vi "testpy.vi"() -> ()   [LabVIEW 2018]
uses:
  <vilib>/Enthought/Python Integration Toolkit/api/Unpack Double.vi
  <vilib>/Enthought/Python Integration Toolkit/Python Integration Toolkit.lvlib
panel:
  out "Value":dbl
  in  "Numeric":dbl format="%#_13g"
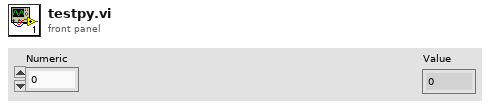
[diagram p1: front panel]
types:
  T1 = typedef "Python Integration Toolkit.lvlib/Session ID.ctl" = u64
  T2 = typedef "Python Integration Toolkit.lvlib/Python Objects.ctl" = variant
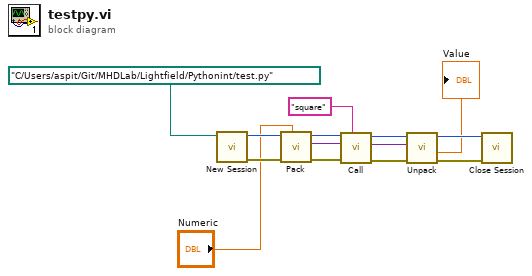
[diagram p0: block diagram]
diagram:
  n1 = call <vilib>:"New Session.vi"("Path to Python Module (.py File)"=path "C:/Users/aspit/Git/MHDLab/Lightfield/Pythonint/test.py") -> ("error out"=w10:errorcluster, "Session ID out"=w14:T1)  [unwired: 9 in]
  n2 = call <vilib>:"Pack.vi"("Argument"="Numeric", "error in (no error)"=w10, "Session ID"=w14) -> ("error out"=w9:errorcluster, "Python Object References Out"=w3:T2, "Session ID out"=w13:T1)  [unwired: 6 in]
  n3 = call <vilib>:"Call.vi"("Function or Method Name"="square", "error in (no error)"=w9, "Python Object References In"=w3, "Session ID"=w13) -> ("error out"=w8:errorcluster, "Python Object References Out"=w2:T2, "Session ID out"=w12:T1)  [unwired: 5 in]
  n4 = call-poly <vilib>:"Unpack.vi"("error in (no error)"=w8, "Python Object References In"=w2, "Session ID"=w12) -> ("error out"=w7:errorcluster, "Value"=→"Value":dbl, "Session ID out"=w11:T1)  [unwired: 5 in, 1 out]
  n5 = call <vilib>:"Close Session.vi"("error in (no error)"=w7, "Session ID"=w11) -> ()  [unwired: 9 in, 1 out]
